vi "IsIntU64.vi"(4 "x":u64) -> (1 "Integer?":bool)   [LabVIEW 2017, in "GPComparison.lvlib"]
doc: "<B>Integer?</B> will be True if <B>x</B> is an integer.\n\nThis VI is inlined.\n\nSteen Schmidt\nGPower\n6/3 2013"
uses:
  GPComparison.lvlib
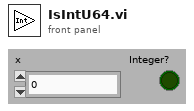
[diagram p1: front panel]
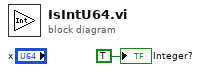
[diagram p0: block diagram]
diagram:
  "Integer?" <- TRUE ("Integer?")
